vi "Analyze Imaq Image.vi"(8 "error in (no error)":errorcluster, 10 "imaq image ref":T1, 11 "transformCvToolkit in":refnum<class "transformCvToolkit.lvclass">) -> (0 "error out":errorcluster, 3 "transformCvToolkit out":refnum<class "transformCvToolkit.lvclass">)   [LabVIEW 2024, in "transformCvToolkit.lvclass"]
uses:
  transformCvToolkit.lvclass
  transformCvToolkit.lvclass/transformCvToolkit.ctl
  <vilib>/vision/Image Controls.llb/IMAQ Image.ctl
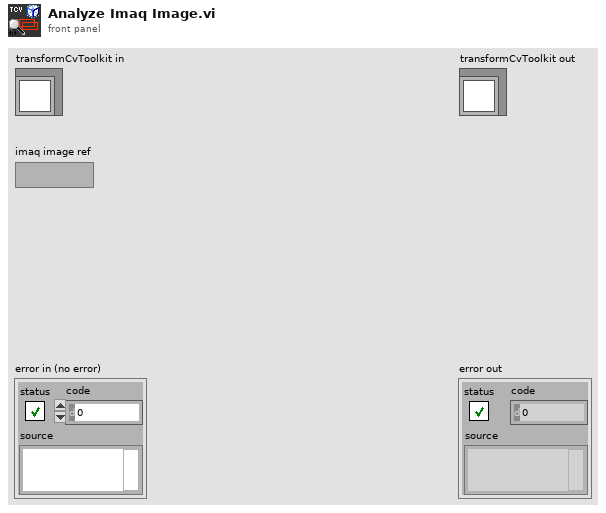
[diagram p1: front panel]
types:
  T1 = typedef "IMAQ Image.ctl" = refnum<image>
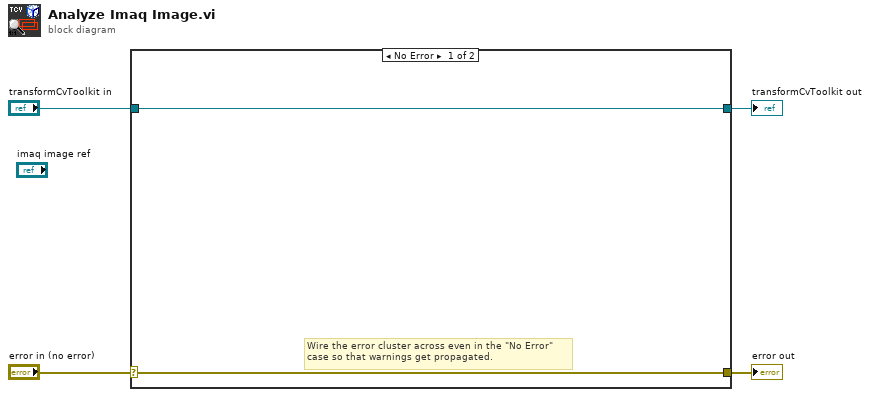
[diagram p0: block diagram]
diagram:
  n1 = case shown="No Error" "error in (no error)" {
    selector: "error in (no error)" -> [w5 w8]
    tunnel: [w5 w8] -> w3
    tunnel: [w6 w7] -> w1
    tunnel: "transformCvToolkit in" -> [w6 w7]
    frame No Error {
      # "Wire the error cluster across even in the \"No Error\"\ncase so that warnings get propagated."
    }
    frame Error {
    }
  }
  "error out" <- w3
  "transformCvToolkit out" <- w1
